vi "Fetch Task from Map.vi"(0 "Task map in":map{string, refnum<k21>}(c390), 5 "Task in":refnum<k21>, 11 "error in (no error)":errorcluster) -> (4 "Task out":refnum<k21>, 15 "error out":errorcluster)   [LabVIEW 2021, in "NI DAQmx_wrapper.lvlib"]
uses:
  NI DAQmx_wrapper.lvlib
  <vilib>/Utility/error.llb/Error Cluster From Error Code.vi
  <vilib>/ErrorRing/Error Ring.xnode
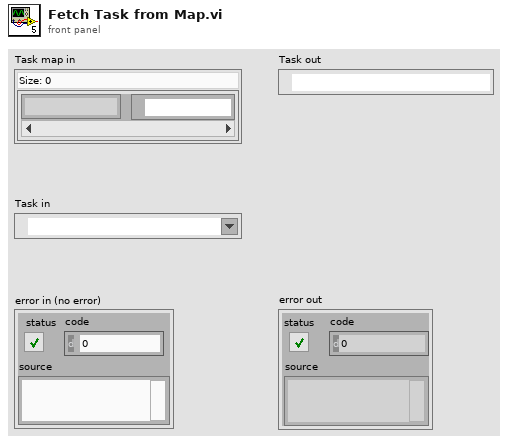
[diagram p1: front panel]
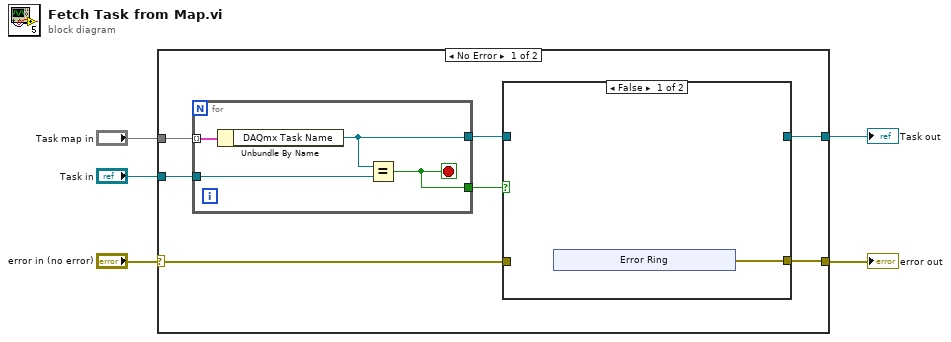
[diagram p0: block diagram]
diagram:
  n1 = case shown="No Error" "error in (no error)" {
    selector: "error in (no error)" -> [w8 w25]
    tunnel: "Task map in" -> [w12 _]
    tunnel: [w6 _] -> w3
    tunnel: [w7 w25] -> w2
    tunnel: "Task in" -> [w11 _]
    frame No Error {
      n2 = for {
        tunnel: w12 -> [w24] mode=indexing
        tunnel: w11 -> [w23]
        tunnel: [w22] -> w9
        tunnel: [w21] -> w10
        stop <- w21 stop-if-true
        n3 = Unbundle By Name(w24) -> ("DAQmx Task Name"=w22:refnum<k21>)
        n4 = Equal?(x=w22, y=w23) -> (x = y?=w21:bool)
      }
      n5 = case shown="False" w10 {
        tunnel: w9 -> [_ w19]
        tunnel: w8 -> [_ w20]
        tunnel: [w13 w20] -> w7
        tunnel: [_ w19] -> w6
        frame False {
          n6 = xnode "Error Ring"() -> ("error out"=w13:errorcluster)
        }
        frame True {
        }
      }
    }
    frame Error {
    }
  }
  "Task out" <- w3
  "error out" <- w2
